vi "VolClockGen.vi"(8 "Num Slices":u16, 11 "Frame Clk In":bool) -> (0 "Volume Clk Out":bool, 4 "Pulse Start":bool)   [LabVIEW 2015]
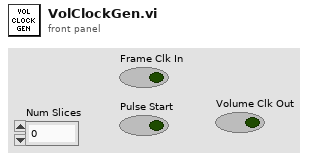
[diagram p1: front panel]
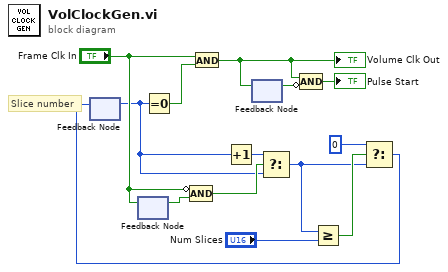
[diagram p0: block diagram]
diagram:
  # "Slice number"
  n1 = feedback #1() -> (w7:u16)  [unwired: 1 in]
  n2 = feedback #2() -> (w11:bool)  [unwired: 1 in]
  n3 = feedback-in #2("Frame Clk In") -> ()
  n4 = Equal To 0?(x=w7) -> (x = 0?=w6:bool)
  n5 = Compound Arithmetic op=AND(invert "Frame Clk In", w11) -> (w9:bool)
  n6 = And(x="Frame Clk In", y=w6) -> (x .and. y?=w13:bool)
  "Volume Clk Out" <- w13
  n7 = Increment(x=w7) -> (x+1=w8:u16)
  n8 = feedback #3() -> (w14:bool)  [unwired: 1 in]
  n9 = feedback-in #3(w13) -> ()
  n10 = Select(t=w8, s=w9, f=w7) -> (s? t:f=w2:u16)
  n11 = Compound Arithmetic op=AND(w13, invert w14) -> (→"Pulse Start":bool)
  n12 = Greater Or Equal?(x=w2, y="Num Slices") -> (x >= y?=w3:bool)
  n13 = Select(t=u16 0, s=w3, f=w2) -> (s? t:f=w5:u16)
  n14 = feedback-in #1(w5) -> ()
